vi "Create Array Of Simple Arithmetic Class Instances.vi"() -> (3 "output array":refnum<class "SimpleArithmetic.lvclass">[](array[class]))   [LabVIEW 2011]
uses:
  ClassDefinitions/SimpleClassWithMethods/SimpleArithmetic.lvclass
panel:
  in  "Array":refnum<class "SimpleArithmetic.lvclass">[](array[class])
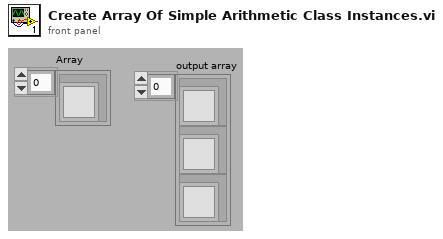
[diagram p1: front panel]
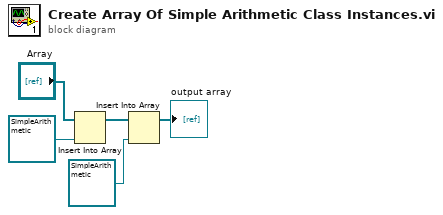
[diagram p0: block diagram]
diagram:
  n1 = Insert Into Array(array="Array", new element=refnum<class "SimpleArithmetic.lvclass"> refnum ("SimpleArithmetic.lvclass")) -> (w4:refnum<class "SimpleArithmetic.lvclass">[])  [unwired: 1 in]
  n2 = Insert Into Array(array=w4, new element=refnum<class "SimpleArithmetic.lvclass"> refnum ("SimpleArithmetic.lvclass")) -> (→"output array":refnum<class "SimpleArithmetic.lvclass">[])  [unwired: 1 in]
